vi "CRYUpdate Edit Step Name.vi"(10 "Proper VI No":u16, 11 "Tree reference In":refnum<vi>) -> (3 "reference out":refnum<vi>)   [LabVIEW 2013]
uses:
  CRYProject Editor Global.vi
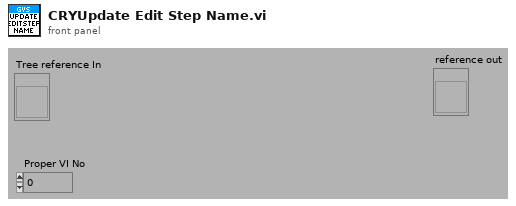
[diagram p1: front panel]
types:
  T1 = typedef "CRYTS.ctl" = cluster{"No.TS":u16, "TS File Path":path, "TS Name":string, "EditStepName":string, "Steps":T2[], "New State":bool, "Change State":bool, "Flattened CurveLib Data":string, "Document Data":string, "EditStepNo":u16, "Operator Start File":string, "Sequence Type":string, "Sequence Language":string}
  T2 = typedef "CRYStep.ctl" = cluster{"No.VI":i32, "Category":string, "StepName":string, "Seq setup flattened":string, "Comment":string, "Steps config.":bool[], "Jump config":i32[], "Start":dbl, "Increment":dbl, "Name":string, "Unit":string, "Y data":u16, "Y prefix":string, "Y dB ref":dbl, "Y unit":string, "Repeat State Array":cluster{"Start":dbl, "Increment":dbl, "Count":i32, "Num":i32}[]}
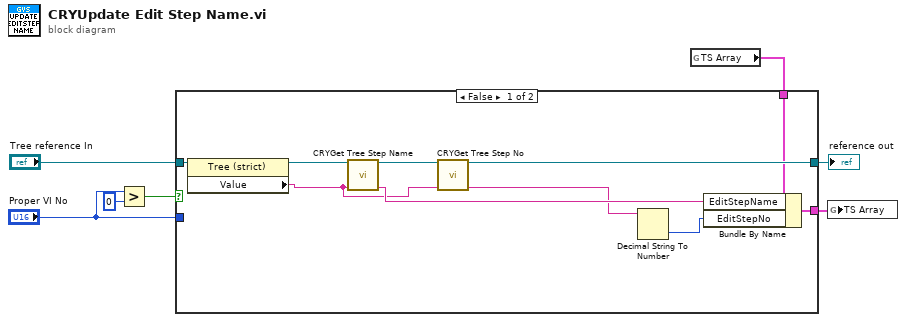
[diagram p0: block diagram]
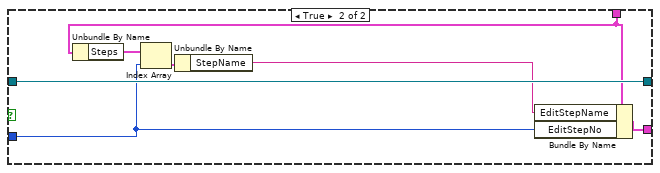
[diagram p2: hidden frame]
diagram:
  n1 = Greater?(x="Proper VI No", y=u16 0) -> (0:w3:bool)
  n2 = global read "CRYProject Editor Global.vi" "TS Array"() -> (w4:T1)
  n3 = case shown="False" w3 {
    tunnel: "Tree reference In" -> [w17 w23]
    tunnel: [w16 w24] -> w6
    tunnel: [w9 w23] -> w5
    tunnel: w4 -> [w8 w22]
    tunnel: "Proper VI No" -> [_ w18]
    frame False {
      n4 = property on="Property Node" class="Tree (strict)"(reference=w17) -> (reference out=w14:refnum<vi>, "Value"=w11:string)  [unwired: 1 in, 1 out]
      n5 = call "CRYGet Tree Step Name.vi"("SequenceTree"=w14, "Active Item Tag"=w11) -> ("reference out"=w12:refnum<vi>, "Active Cell String0"=w13:string)  [unwired: 12 in]
      n6 = call "CRYGet Tree Step No.vi"("SequenceTree"=w12, "Active Item Tag"=w11) -> ("reference out"=w9:refnum<vi>, "Active Cell String4"=w10:string)  [unwired: 12 in]
      n7 = Decimal String To Number(string=w10) -> (number=w15:i32)  [unwired: 2 in, 1 out]
      n8 = Bundle By Name(cluster=w8, "EditStepName"=w13, "EditStepNo"=w15) -> (w16:T1)
    }
    frame True {
      n9 = Unbundle By Name(w22) -> ("Steps"=w21:T2[])
      n10 = Index Array(array=w21, index=w18) -> (element=w20:T2)
      n11 = Unbundle By Name(w20) -> ("StepName"=w19:string)
      n12 = Bundle By Name(cluster=w22, "EditStepName"=w19, "EditStepNo"=w18) -> (w24:T1)
    }
  }
  "reference out" <- w5
  n13 = global write "CRYProject Editor Global.vi" "TS Array"(w6) -> ()
